vi "thorlabs_query_positions.vi"(8 "error in (no error)":errorcluster, 11 "thorlabs_panel in":refnum<class "thorlabs_panel.lvclass">) -> (0 "error out":errorcluster, 3 "thorlabs_panel out":refnum<class "thorlabs_panel.lvclass">)   [LabVIEW 2015, in "thorlabs_panel.lvclass"]
uses:
  thorlabs_panel.lvclass
  thorlabs_class/thorlabs_kinesis.lvclass
  thorlabs_panel.lvclass/thorlabs_panel.ctl
  UI/panel_class/panel.lvclass
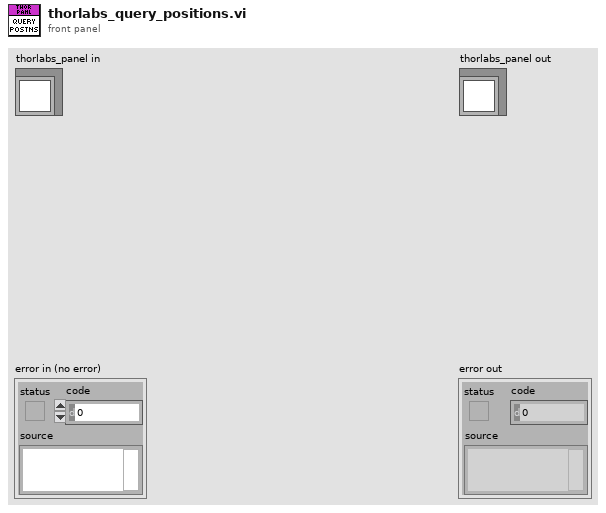
[diagram p1: front panel]
types:
  T1 = typedef "thorlabs_events.ctl" = cluster{"mcl_status":refnum<user-event>, "piezo_positions":refnum<user-event>}
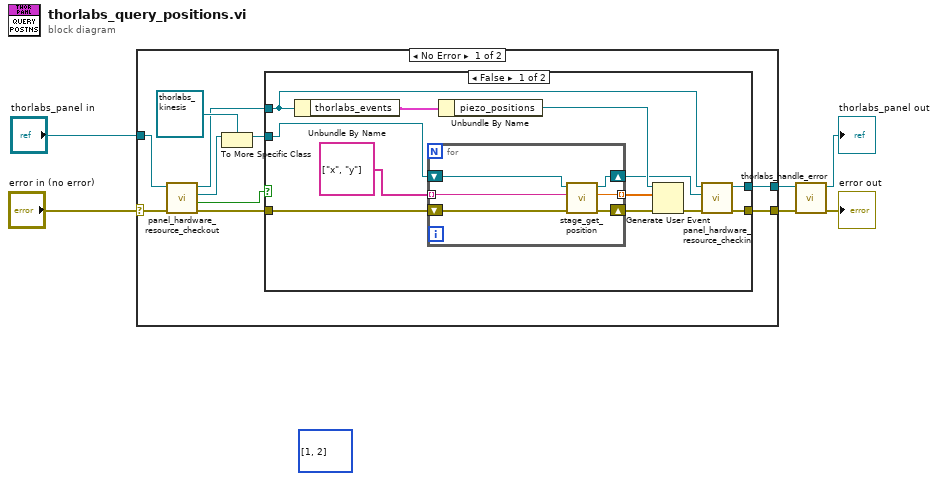
[diagram p0: block diagram]
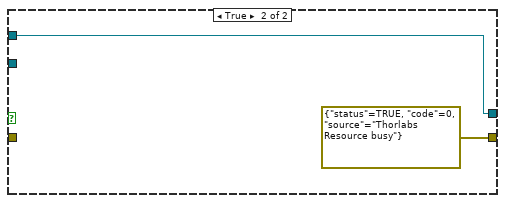
[diagram p2: hidden frame]
diagram:
  (unwired) i32[] [1, 2]
  n1 = case shown="No Error" "error in (no error)" {
    selector: "error in (no error)" -> [w15 w38]
    tunnel: [w7 w38] -> w1
    tunnel: "thorlabs_panel in" -> [w16 w37]
    tunnel: [w8 w37] -> w3
    frame No Error {
      n2 = call "panel_hardware_resource_checkout.vi"("error in (no error)"=w15, "panel in"=w16) -> ("error out"=w11:errorcluster, "timed out?"=w10:bool, "hardware.lvclass"=w14:refnum<class "hardware.lvclass">, "panel out"=w9:refnum<class "thorlabs_panel.lvclass">)  [unwired: 6 in]
      n3 = To More Specific Class(target class=refnum<class "thorlabs_kinesis.lvclass"> refnum ("thorlabs_kinesis.lvclass"), reference=w14) -> (specific class reference=w12:refnum<class "thorlabs_kinesis.lvclass">)  [unwired: 1 in, 1 out]
      n4 = case shown="False" w10 {
        tunnel: w12 -> [w26 _]
        tunnel: w11 -> [w25 _]
        tunnel: w9 -> [w24 w35]
        tunnel: [w28 w35] -> w8
        tunnel: [w27 errorcluster {"status"=TRUE, "code"=0, "source"="Thorlabs Resource busy"} ("error out")] -> w7
        frame False {
          n5 = Unbundle By Name(w24) -> ("thorlabs_events"=w23:T1)
          n6 = for {
            shift-right: [w33] -> w18
            shift-left: w25 -> [w34]
            shift-right: [w31] -> w19
            shift-left: w26 -> [w32]
            tunnel: string[] ["x", "y"] -> [w30] mode=indexing
            tunnel: [w29] -> w21 mode=indexing
            n7 = call-dynamic "stage_get_position.vi"("error in (no error)"=w34, "Stage Name"=w30, "Stage in"=w32) -> ("error out"=w33:errorcluster, "Position"=w29:dbl, "Stage out"=w31:refnum<class "thorlabs_kinesis.lvclass">)  [unwired: 6 in]
          }
          n8 = Unbundle By Name(w23) -> ("piezo_positions"=w22:refnum<user-event>)
          n9 = Generate User Event(user event=w22, event data cluster=w21, error in=w18) -> (error out=w20:errorcluster)  [unwired: 1 in, 1 out]
          n10 = call "panel_hardware_resource_checkin.vi"("error in (no error)"=w20, "hardware.lvclass"=w19, "panel in"=w24) -> ("error out"=w27:errorcluster, "panel out"=w28:refnum<class "thorlabs_panel.lvclass">)  [unwired: 7 in]
        }
        frame True {
        }
      }
    }
    frame Error {
    }
  }
  n11 = call "thorlabs_handle_error.vi"("error in (no error)"=w1, "thorlabs_panel in"=w3) -> ("error out"=→"error out":errorcluster, "thorlabs_panel out"=→"thorlabs_panel out":refnum<class "thorlabs_panel.lvclass">)  [unwired: 8 in]
